vi "Toggle2.vi"(1 "Boolean 2":bool, 2 "Boolean":bool) -> (0 "Numeric":dbl)   [LabVIEW 2017]
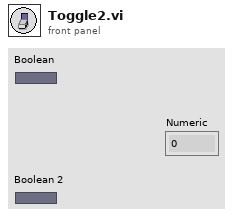
[diagram p1: front panel]
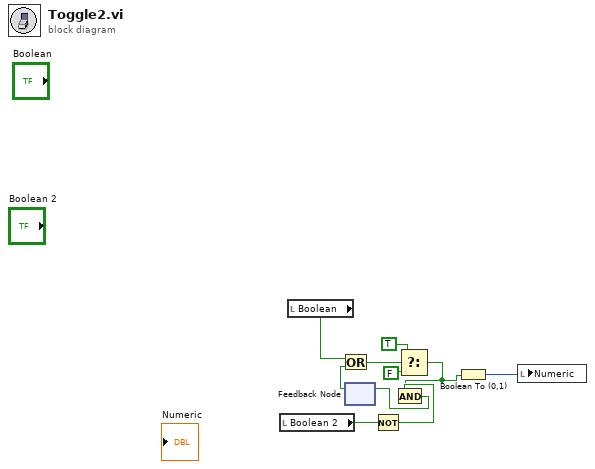
[diagram p0: block diagram]
diagram:
  n1 = local read "Boolean 2"() -> (w3:bool)
  n2 = local read "Boolean"() -> (w4:bool)
  n3 = feedback #1() -> (w5:bool)  [unwired: 1 in]
  n4 = Or(x=w4, y=w5) -> (x .or. y?=w8:bool)
  n5 = Not(x=w3) -> (.not. x?=w7:bool)
  n6 = Select(t=TRUE, s=w8, f=FALSE) -> (s? t:f=w2:bool)
  n7 = And(x=w2, y=w7) -> (x .and. y?=w6:bool)
  n8 = feedback-in #1(w6) -> ()
  n9 = Boolean To (0,1)(Boolean=w2) -> (0, 1=w1:i16)
  n10 = local write "Numeric"(w1) -> ()
